vi "Acquire Continuously.vi"(8 "error in (no error)":errorcluster, 11 "Strain in":refnum<class "Strain.lvclass">) -> (0 "error out":errorcluster, 3 "Strain out":refnum<class "Strain.lvclass">)   [LabVIEW 2015, in "Strain.lvlib" / "Strain.lvclass"]
uses:
  Strain.lvclass
  <userlib>/Common Components/Measurement Actor/Measurement.lvclass
  <vilib>/measure/NI_MABase.lvlib
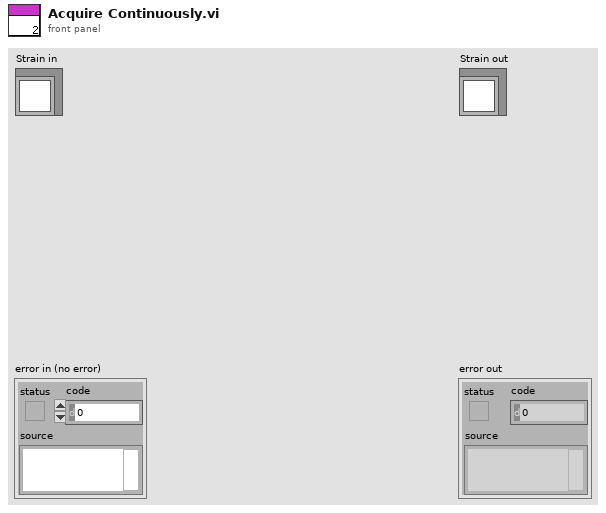
[diagram p1: front panel]
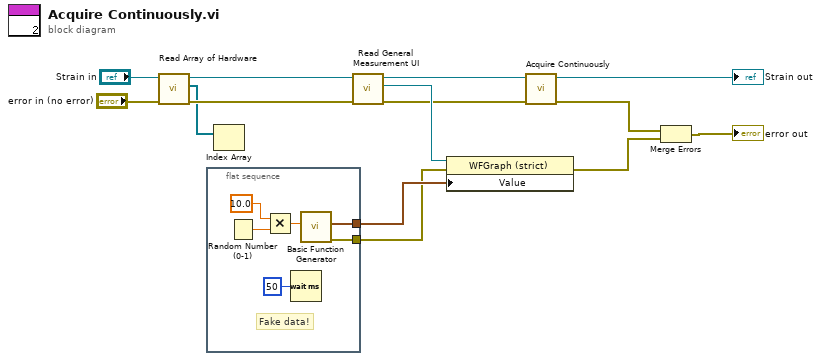
[diagram p0: block diagram]
diagram:
  n1 = call <userlib>:"Read Array of Hardware.vi"("error in (no error)"="error in (no error)", "Measurement in"="Strain in") -> ("error out"=w7:errorcluster, "Array of Hardware"=w1:refnum<class "Hardware.lvclass">[], "Measurement out"=w9:refnum<class "Strain.lvclass">)  [unwired: 7 in]
  n2 = flat-sequence {
    tunnel: [w17] -> w12
    tunnel: [w15] -> w5
    frame #0 {
      # "Fake data!"
      n3 = Random Number (0-1)() -> (number: 0 to 1=w18:dbl)
      n4 = Multiply(x=10.0, y=w18) -> (x*y=w20:dbl)
      n5 = Wait (ms)(milliseconds to wait=u32 50) -> ()  [unwired: 1 out]
      n6 = call <vilib>:"Basic Function Generator.vi"("amplitude"=w20) -> ("error out"=w15:errorcluster, "signal out"=w17:waveform(dbl))  [unwired: 8 in, 1 out]
    }
  }
  n7 = Index Array(array=w1) -> ()  [unwired: 1 in, 1 out]
  n8 = call <userlib>:"Read General Measurement UI.vi"("error in (no error)"=w7, "Measurement in"=w9) -> ("error out"=w6:errorcluster, "General Measurement UI"=w13:refnum<vi>, "Measurement out"=w11:refnum<class "Strain.lvclass">)  [unwired: 7 in]
  n9 = property class="WFGraph (strict)"(reference=w13, error in=w5, "Value"=w12) -> (error out=w4:errorcluster)  [unwired: 1 out]
  n10 = call-parent "Acquire Continuously.vi"("error in (no error)"=w6, "Measurement in"=w11) -> ("error out"=w3:errorcluster, "Measurement out"=→"Strain out":refnum<class "Strain.lvclass">)  [unwired: 8 in]
  n11 = Merge Errors(w3, w4) -> (→"error out":errorcluster)
